vi "Motors Redefine Origin Bk.vi"(2 "error in":errorcluster, 3 "VISA in":refnum<visa-resource-name>) -> (0 "error out":errorcluster, 1 "VISA out":refnum<visa-resource-name>)   [LabVIEW 2010]
panel:
  out "CP 1":string
  out "CP 2":string
  out "CP 3":string
  out "CP 4":string
  out "AP 4":string
  out "AP 3":string
  out "AP 2":string
  out "AP 1":string
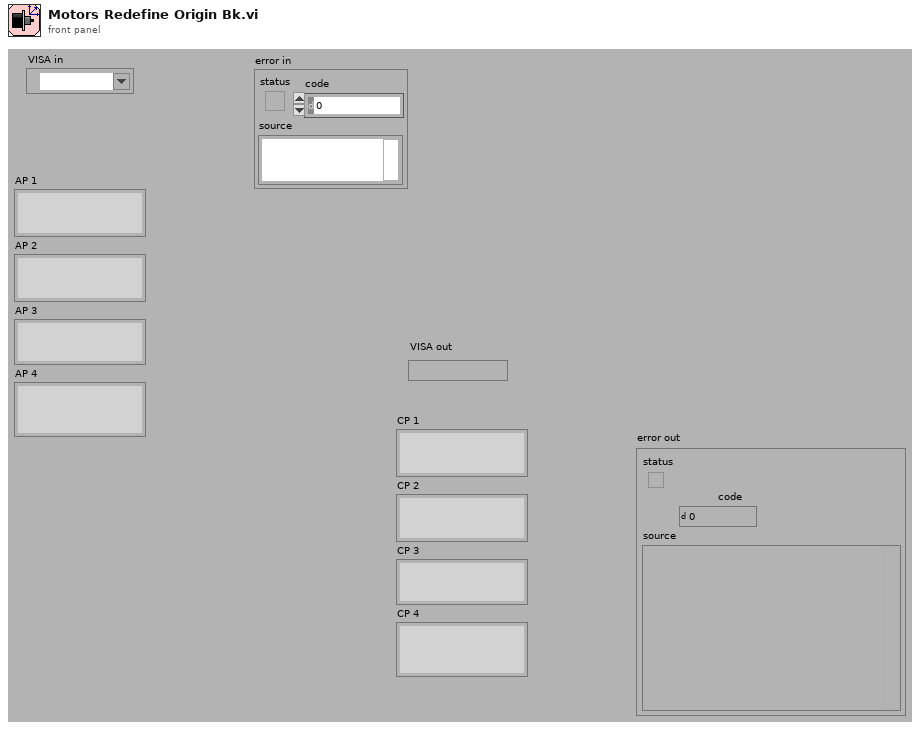
[diagram p1: front panel]
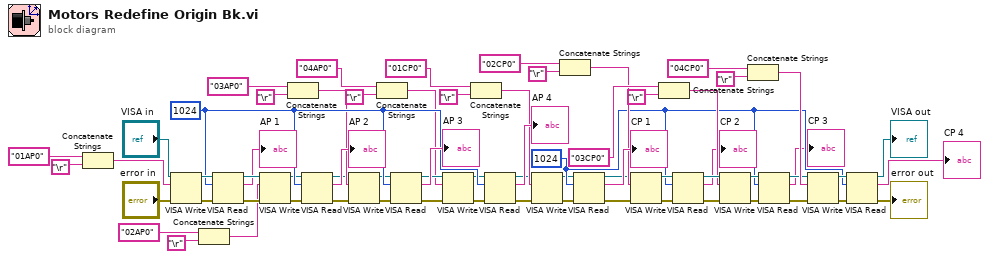
[diagram p0: block diagram]
diagram:
  w13 = u32 1024 ("byte count")
  w60 = u32 1024 ("byte count")
  n1 = Concatenate Strings("01AP0" ("Initial command 1"), "\r") -> (w66:string)
  n2 = VISA Write(VISA resource name="VISA in", write buffer=w66, error in (no error)="error in") -> (VISA resource name out=w64:refnum<visa-resource-name>, error out=w65:errorcluster)  [unwired: 1 out]
  n3 = Concatenate Strings("02AP0" ("Initial command 2"), "\r") -> (w53:string)
  n4 = VISA Read(VISA resource name=w64, byte count=w60, error in (no error)=w65) -> (VISA resource name out=w59:refnum<visa-resource-name>, read buffer=→"AP 1":string, error out=w58:errorcluster)  [unwired: 1 out]
  n5 = VISA Write(VISA resource name=w59, write buffer=w53, error in (no error)=w58) -> (VISA resource name out=w57:refnum<visa-resource-name>, error out=w56:errorcluster)  [unwired: 1 out]
  n6 = Concatenate Strings("03AP0" ("Initial command 3"), "\r") -> (w50:string)
  n7 = VISA Read(VISA resource name=w57, byte count=w60, error in (no error)=w56) -> (VISA resource name out=w48:refnum<visa-resource-name>, read buffer=→"AP 2":string, error out=w49:errorcluster)  [unwired: 1 out]
  n8 = VISA Write(VISA resource name=w48, write buffer=w50, error in (no error)=w49) -> (VISA resource name out=w46:refnum<visa-resource-name>, error out=w47:errorcluster)  [unwired: 1 out]
  n9 = Concatenate Strings("04AP0" ("Initial command 4"), "\r") -> (w40:string)
  n10 = VISA Read(VISA resource name=w46, byte count=w60, error in (no error)=w47) -> (VISA resource name out=w45:refnum<visa-resource-name>, read buffer=→"AP 3":string, error out=w44:errorcluster)  [unwired: 1 out]
  n11 = VISA Write(VISA resource name=w45, write buffer=w40, error in (no error)=w44) -> (VISA resource name out=w42:refnum<visa-resource-name>, error out=w43:errorcluster)  [unwired: 1 out]
  n12 = Concatenate Strings("01CP0" ("Initial command 1"), "\r") -> (w5:string)
  n13 = VISA Read(VISA resource name=w42, byte count=w60, error in (no error)=w43) -> (VISA resource name out=w2:refnum<visa-resource-name>, read buffer=→"AP 4":string, error out=w1:errorcluster)  [unwired: 1 out]
  n14 = VISA Write(VISA resource name=w2, write buffer=w5, error in (no error)=w1) -> (VISA resource name out=w9:refnum<visa-resource-name>, error out=w8:errorcluster)  [unwired: 1 out]
  n15 = Concatenate Strings("02CP0" ("Initial command 2"), "\r") -> (w20:string)
  n16 = VISA Read(VISA resource name=w9, byte count=w13, error in (no error)=w8) -> (VISA resource name out=w14:refnum<visa-resource-name>, read buffer=→"CP 1":string, error out=w15:errorcluster)  [unwired: 1 out]
  n17 = VISA Write(VISA resource name=w14, write buffer=w20, error in (no error)=w15) -> (VISA resource name out=w16:refnum<visa-resource-name>, error out=w17:errorcluster)  [unwired: 1 out]
  n18 = Concatenate Strings("03CP0" ("Initial command 3"), "\r") -> (w23:string)
  n19 = VISA Read(VISA resource name=w16, byte count=w13, error in (no error)=w17) -> (VISA resource name out=w25:refnum<visa-resource-name>, read buffer=→"CP 2":string, error out=w24:errorcluster)  [unwired: 1 out]
  n20 = VISA Write(VISA resource name=w25, write buffer=w23, error in (no error)=w24) -> (VISA resource name out=w27:refnum<visa-resource-name>, error out=w26:errorcluster)  [unwired: 1 out]
  n21 = Concatenate Strings("04CP0" ("Initial command 4"), "\r") -> (w33:string)
  n22 = VISA Read(VISA resource name=w27, byte count=w13, error in (no error)=w26) -> (VISA resource name out=w28:refnum<visa-resource-name>, read buffer=→"CP 3":string, error out=w29:errorcluster)  [unwired: 1 out]
  n23 = VISA Write(VISA resource name=w28, write buffer=w33, error in (no error)=w29) -> (VISA resource name out=w31:refnum<visa-resource-name>, error out=w30:errorcluster)  [unwired: 1 out]
  n24 = VISA Read(VISA resource name=w31, byte count=w13, error in (no error)=w30) -> (VISA resource name out=→"VISA out":refnum<visa-resource-name>, read buffer=→"CP 4":string, error out=→"error out":errorcluster)  [unwired: 1 out]
